vi "Execute Script.vi"(4 "ms timeout (-1)":i32=-1, 6 "Name":string="script", 7 "Script":string, 8 "error in":errorcluster, 10 "Argument Data":variant, 11 "GLue in":refnum<class "class.GLue.lvclass">) -> (0 "error out":errorcluster, 2 "Return Data":variant, 3 "GLue out":refnum<class "class.GLue.lvclass">)   [LabVIEW 2014, in "GLue.lvlib"]
doc: "Executes a provided Lua script.\n\n<B>Parameter(s) </B>\n-----------------\n\n- <B>GLue in:</B> Reference to the GLue instance.\n\n- <B>Script:</B> Lua script to be executed.\n\n- <B>Name:</B> Name of the provided script.\n\n- <B>Argument Data:</B> LabVIEW variant used as argument data for the Lua script.\n\n- <B>ms timeout (-1):</B> The time to wait for the GLue reference to become available. A value of '-1' specifies an infinite timeout.\n\n- <B>error in:</B> Describes error conditions that occur before this VI runs. This input provides standard error in functionality. \n\n- <B>GLue out:</B> Reference to the GLue instance.\n\n- <B>Return Data:</B> Return data from the Lua script in the form of a LabVIEW variant\n\n- <B>error out:</B> Contains error information. This output provides standard error out functionality."
uses:
  GLue.lvlib
  Private/Class/class.GLue.lvclass
  Private/Class/class.GLue.lvclass/class.GLue.ctl
  <vilib>/Utility/semaphor.llb/Acquire Semaphore.vi
  Private/Class/meth.RunChunk.vi
  <vilib>/Utility/semaphor.llb/Release Semaphore.vi
panel:
  # "Input"
  # "Output"
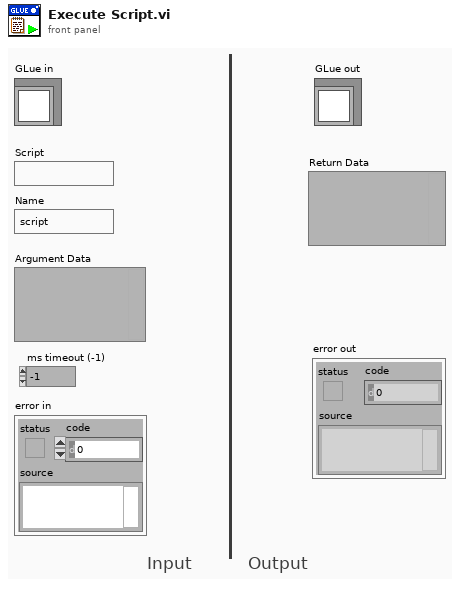
[diagram p1: front panel]
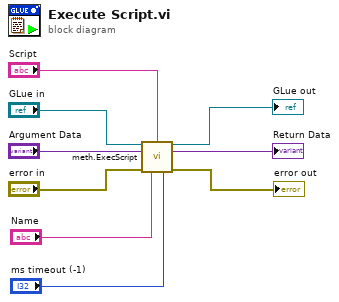
[diagram p0: block diagram]
diagram:
  n1 = call "meth.ExecScript.vi"("GLue in"="GLue in", "Script"="Script", "Argument"="Argument Data", "error in"="error in", "Name"="Name", "ms timeout (-1)"="ms timeout (-1)") -> ("GLue out"=→"GLue out":refnum<class "class.GLue.lvclass">, "Return"=→"Return Data":variant, "error out"=→"error out":errorcluster)  [unwired: 7 in]
